vi "stepper controller -- IMS -- V3.vi"(7 "stepper driver action":T3, 8 "internal stepper driver state IMS":T1={"VISA address"="GPIB0::25::INSTR", "stepper motor state"=enum."stopped", "Motor Address"=0, "speed"=0, "target position"=0.0, "current position"=0.0}, 11 "number":dbl format="%#_13g") -> (0 "internal stepper driver state IMS -- OUT":T1={"VISA address"="GPIB0::25::INSTR", "stepper motor state"=enum."stopped", "Motor Address"=0, "speed"=0, "target position"=0.0, "current position"=0.0}, 1 "stepper motor state OUT":T2, 3 "current position":dbl)   [LabVIEW 2018]
uses:
  stepper motor action.ctl
  stepper motor state.ctl
  internal stepper driver state -- IMS.ctl
  Q - not nan -- integer.vi
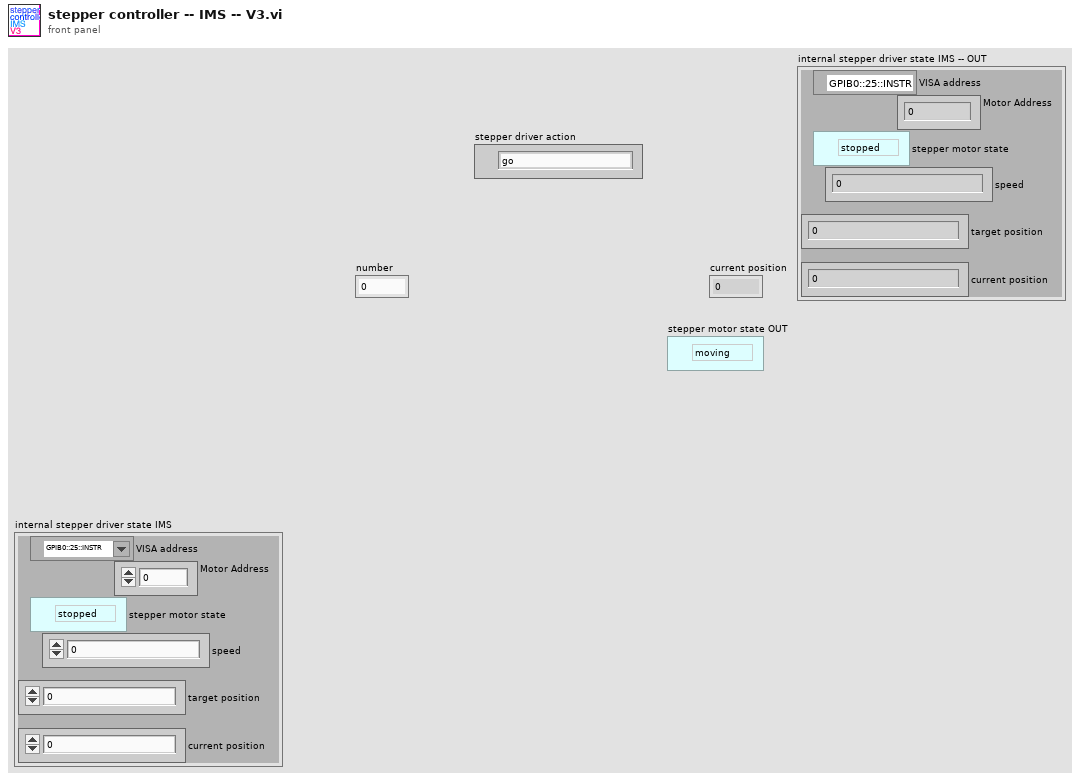
[diagram p1: front panel]
types:
  T1 = typedef "internal stepper driver state -- IMS.ctl" = cluster{"VISA address":refnum<visa-resource-name>, "stepper motor state":T2, "Motor Address":u32, "speed":i32, "target position":dbl, "current position":dbl}
  T2 = typedef "stepper motor state.ctl" = enum16{"moving", "stopped"}
  T3 = typedef "stepper motor action.ctl" = enum16{"go", "void", "stop", "check", "init", "sync", "set", "set speed", "--check status", "--check value"}
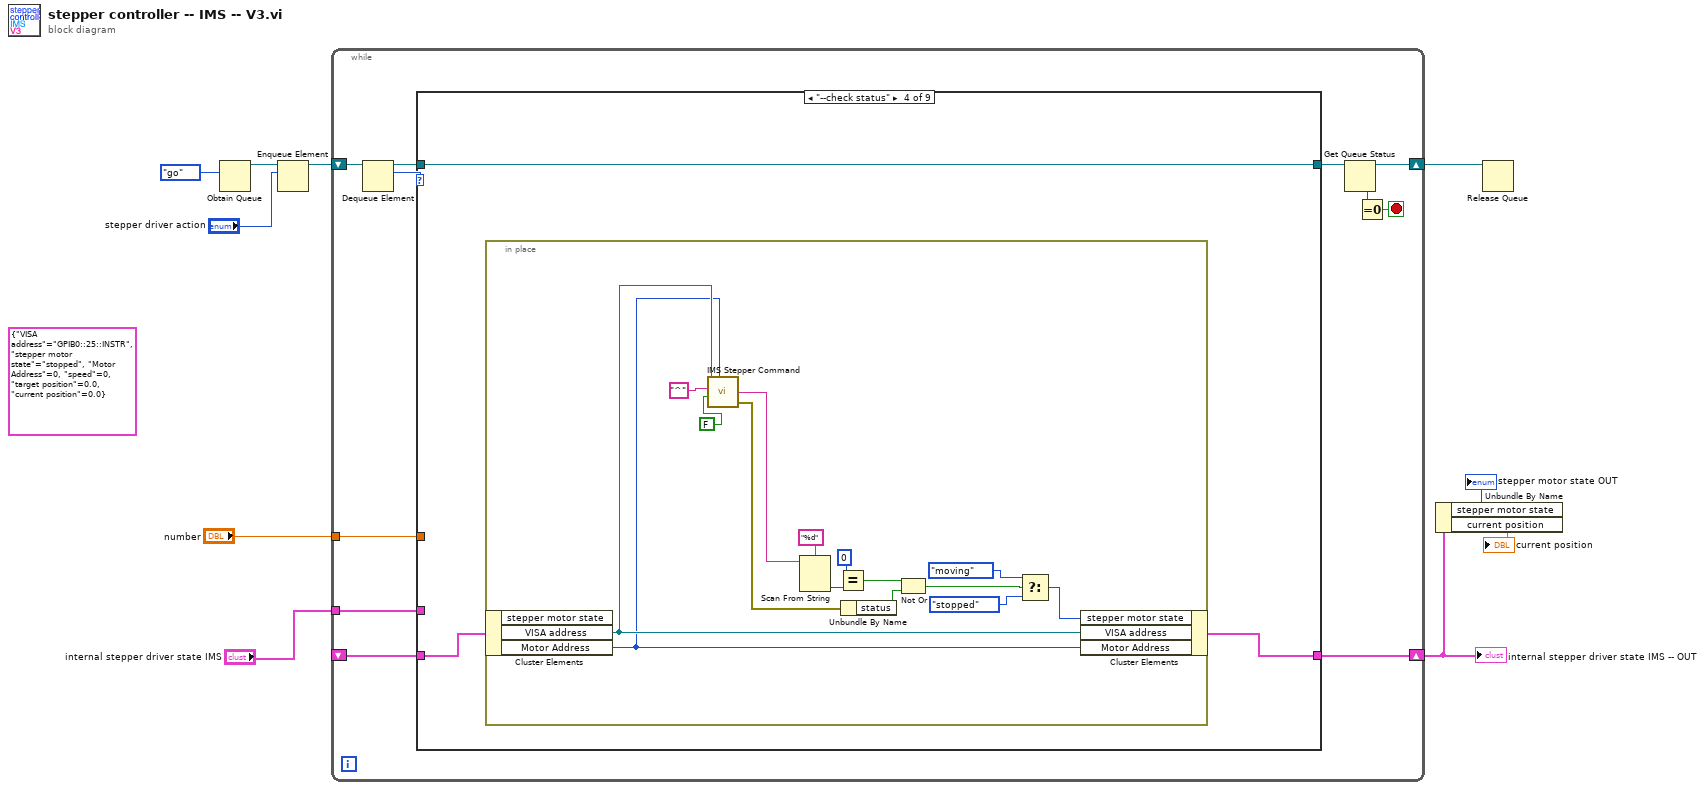
[diagram p0: block diagram]
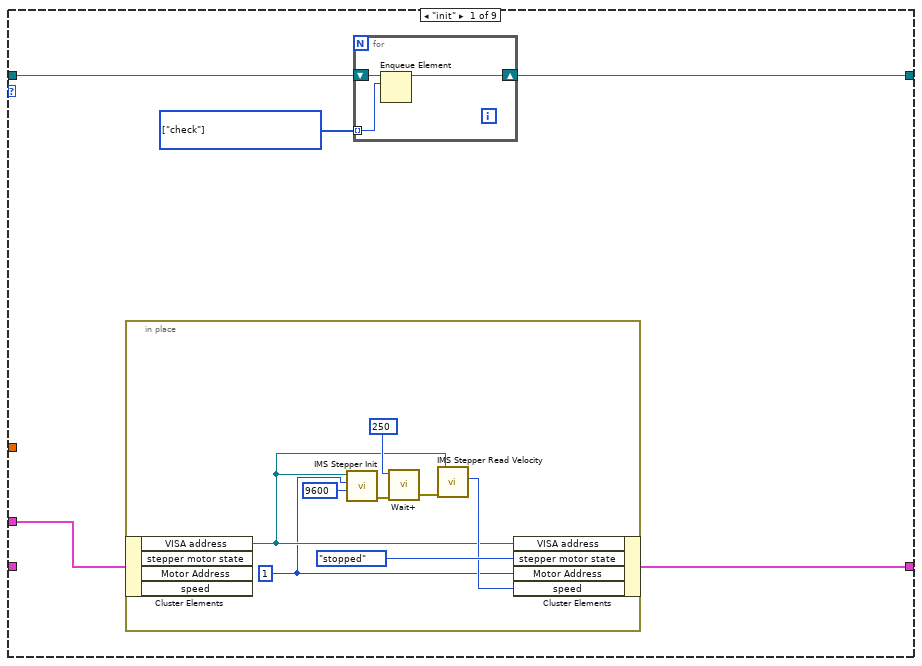
[diagram p2: hidden frame]
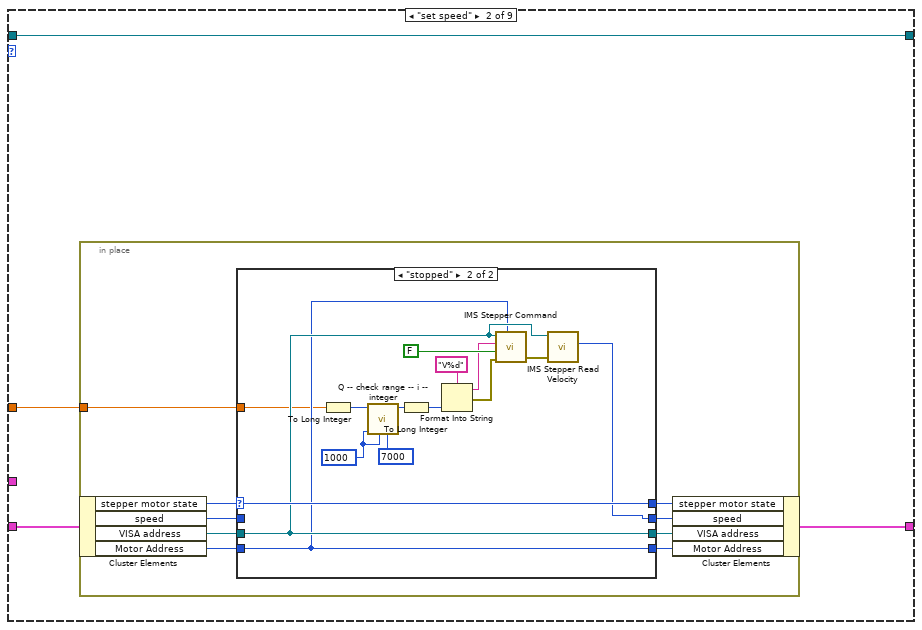
[diagram p3: hidden frame]
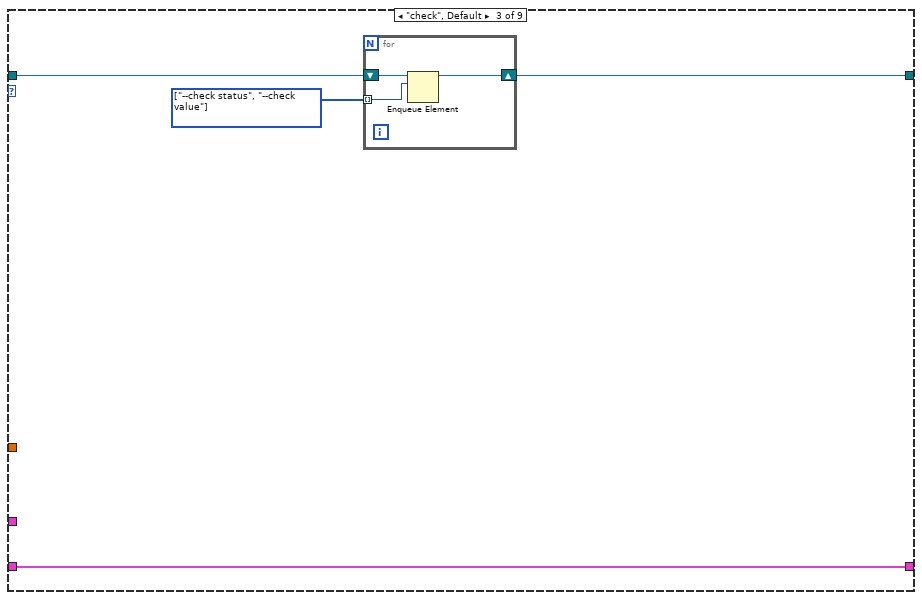
[diagram p5: hidden frame]
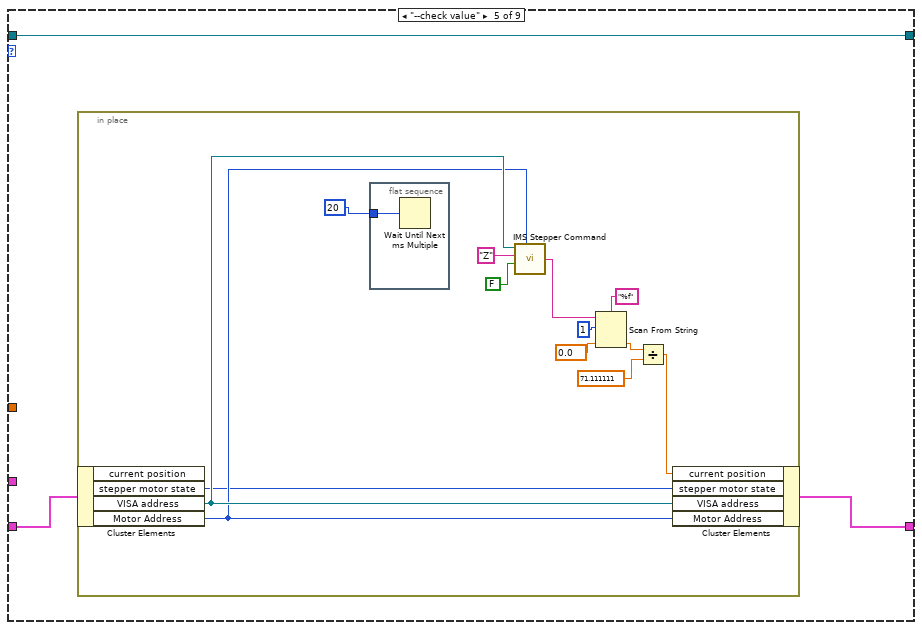
[diagram p6: hidden frame]
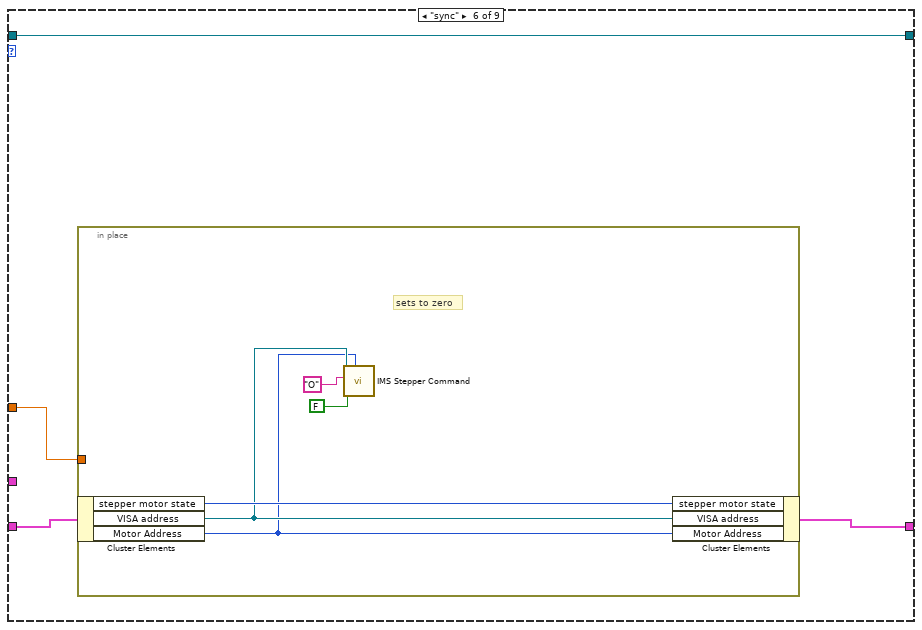
[diagram p7: hidden frame]
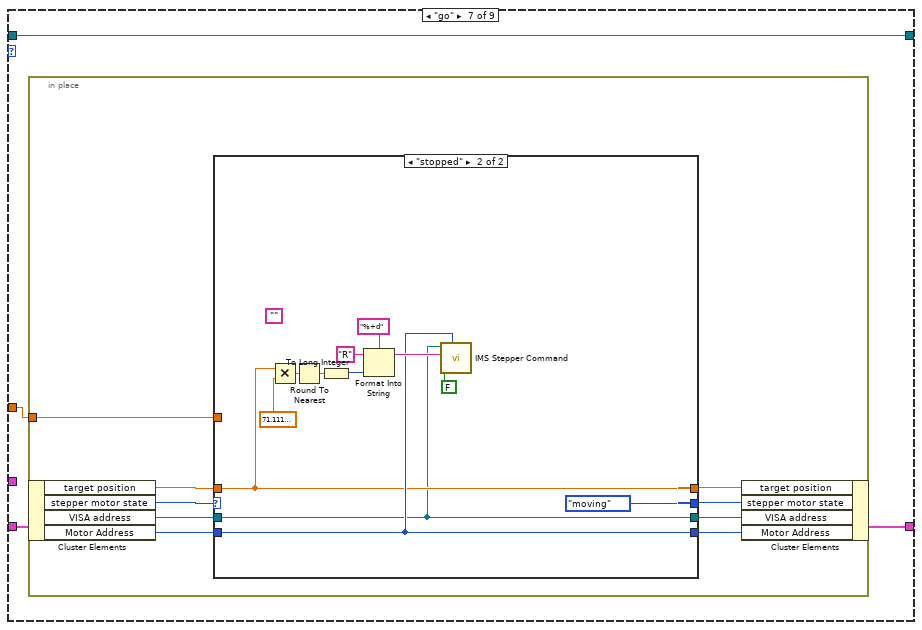
[diagram p8: hidden frame]
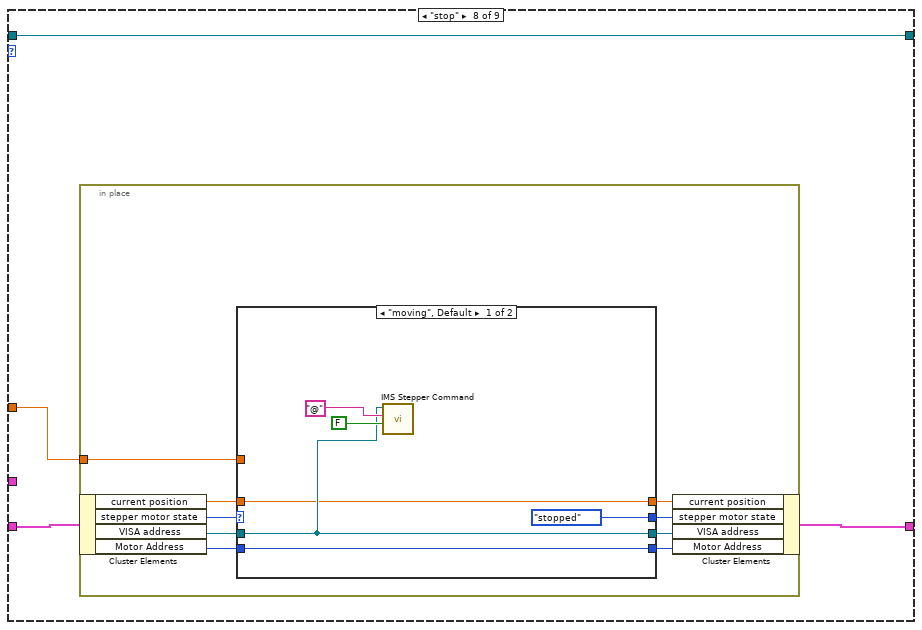
[diagram p10: hidden frame]
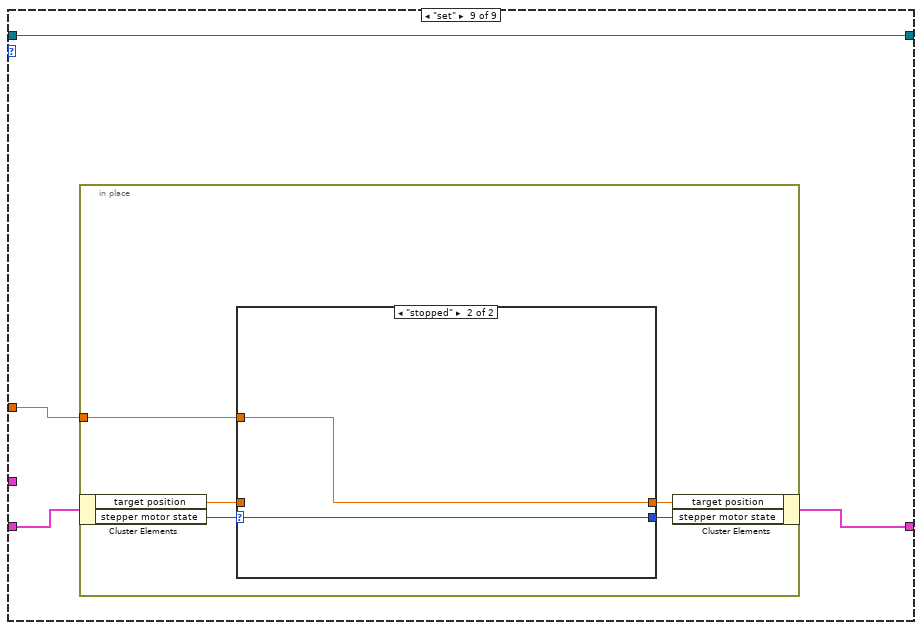
[diagram p12: hidden frame]
diagram:
  (unwired) T1 {"VISA address"="GPIB0::25::INSTR", "stepper motor state"=enum."stopped", "Motor Address"=0, "speed"=0, "target position"=0.0, "current position"=0.0} ("internal stepper driver state IMS")
  n1 = Obtain Queue(element data type=stepper_motor_action."go" ("stepper driver action")) -> (queue out=w4:refnum<queue>)  [unwired: 4 in, 2 out]
  n2 = Enqueue Element(queue=w4, element="stepper driver action") -> (queue out=w3:refnum<queue>)  [unwired: 2 in, 2 out]
  n3 = while {
    shift-right: [w21] -> w6
    shift-left: _ -> [w20]
    shift-right: [w13] -> w1
    shift-left: w3 -> [w17]
    tunnel: "internal stepper driver state IMS" -> [w19]
    tunnel: "number" -> [w18]
    stop <- w11 stop-if-true
    n4 = Dequeue Element(queue=w17) -> (queue out=w16:refnum<queue>, element=w15:T3)  [unwired: 2 in, 2 out]
    n5 = case shown="\"--check status\"" w15 {
      tunnel: [w25 w39 w73 w78 w96 w113 w122 w151 w174] -> w21
      tunnel: w20 -> [_ w40 w73 w79 w97 w114 w123 w152 w175]
      tunnel: [w23 w41 w71 w77 w95 w115 w124 w153 w176] -> w14
      tunnel: w16 -> [w24 w41 w72 w77 w95 w115 w124 w153 w176]
      tunnel: w19 -> [w26 _ _ _ _ _ _ _ _]
      tunnel: w18 -> [_ w38 _ _ _ w112 w121 w150 w173]
      frame "init" {
        w22 = T3[] [enum."check"] items=["go", "void", "stop", "check", "init", "sync", "set", "set speed", "--check status", "--check value"] ("action list IN")
        n6 = in-place {
          w30 = u32 1 ("Motor Address")
          n7 = in-place-cluster #1(w26) -> ("VISA address"=w31:refnum<visa-resource-name>)  [unwired: 3 out]
          n8 = call "IMS Stepper Init.vi"("Baud Rate"=u32 9600, "Motor Number"=w30, "Instrument Address"=w31) -> ("error out"=w36:errorcluster)  [unwired: 1 in, 1 out]
          n9 = call "Wait+.vi"("Error In"=w36, "milliseconds to wait"=u32 250) -> ("Error Out"=w35:errorcluster)  [unwired: 4 in, 1 out]
          n10 = call "IMS Stepper Read Velocity.vi"("error in (no error)"=w35, "Instrument Address"=w31) -> ("Velocity"=w32:i32)  [unwired: 3 in, 2 out]
          n11 = in-place-cluster #1("VISA address"=w31, "stepper motor state"=stepper_motor_state."stopped", "Motor Address"=w30, "speed"=w32) -> (w25:T1)
        }
        n12 = for {
          shift-right: [w28] -> w23
          shift-left: w24 -> [w29]
          tunnel: w22 -> [w27] mode=indexing
          n13 = Enqueue Element(queue=w29, element=w27) -> (queue out=w28:refnum<queue>)  [unwired: 2 in, 2 out]
        }
      }
      frame "set speed" {
        n14 = in-place {
          in-place-border: w38 -> [w50]
          n15 = in-place-cluster #2(w40) -> ("stepper motor state"=w46:T2, "speed"=w45:i32, "VISA address"=w48:refnum<visa-resource-name>, "Motor Address"=w47:u32)
          n16 = case shown="\"stopped\"" w46 {
            selector: w46 -> [w51 w67]
            tunnel: w50 -> [_ w56]
            tunnel: [w54 w58] -> w49
            tunnel: w48 -> [w53 w59]
            tunnel: w47 -> [w52 w57]
            tunnel: w45 -> [w54 _]
            tunnel: [w53 w59] -> w44
            tunnel: [w52 w57] -> w43
            tunnel: [w51 w67] -> w42
            frame "moving", Default {
            }
            frame "stopped" {
              w69 = 1000 ("lower limit")
              n17 = To Long Integer(number=w56) -> (32bit integer=w55:i32)
              n18 = call "Q -- check range -- i -- integer.vi"("upper"=7000 ("x"), "lower"=w69, "default"=w69, "number"=w55) -> ("number in range"=w61:i32)  [unwired: 5 in, 2 out]
              n19 = To Long Integer(number=w61) -> (32bit integer=w60:i32)
              n20 = Format Into String(format string="V%d", w60) -> (resulting string=w64:string, error out=w63:errorcluster)  [unwired: 2 in]
              n21 = call "IMS Stepper Command.vi"("Instrument Address"=w59, "Motor Number"=w57, "Command"=w64, "Mode"=FALSE, "error in (no error)"=w63) -> ("error out"=w62:errorcluster)  [unwired: 1 in, 2 out]
              n22 = call "IMS Stepper Read Velocity.vi"("error in (no error)"=w62, "Instrument Address"=w59) -> ("Velocity"=w58:i32)  [unwired: 3 in, 2 out]
            }
          }
          n23 = in-place-cluster #2("stepper motor state"=w42, "speed"=w49, "VISA address"=w44, "Motor Address"=w43) -> (w39:T1)
        }
      }
      frame "check", Default {
        w70 = T3[] [enum."--check status", enum."--check value"] items=["go", "void", "stop", "check", "init", "sync", "set", "set speed", "--check status", "--check value"] ("action list IN")
        n24 = for {
          shift-right: [w75] -> w71
          shift-left: w72 -> [w76]
          tunnel: w70 -> [w74] mode=indexing
          n25 = Enqueue Element(queue=w76, element=w74) -> (queue out=w75:refnum<queue>)  [unwired: 2 in, 2 out]
        }
      }
      frame "--check status" {
        n26 = in-place {
          n27 = in-place-cluster #3(w79) -> ("VISA address"=w82:refnum<visa-resource-name>, "Motor Address"=w81:u32)  [unwired: 1 out]
          n28 = call "IMS Stepper Command.vi"("Instrument Address"=w82, "Motor Number"=w81, "Command"="^", "Mode"=FALSE) -> ("Response"=w89:string, "error out"=w80:errorcluster)  [unwired: 2 in, 1 out]
          n29 = Scan From String(format string="%d", input string=w89) -> (output 1=w90:i32)  [unwired: 3 in, 3 out]
          n30 = Equal?(x=0, y=w90) -> (x = y?=w91:bool)
          n31 = Unbundle By Name(w80) -> ("status"=w92:bool)
          n32 = Not Or(1:w92, 2:w91) -> (0:w84:bool)
          n33 = Select(t=stepper_motor_state."moving" ("stepper motor state"), s=w84, f=stepper_motor_state."stopped" ("stepper motor state")) -> (s? t:f=w83:T2)
          n34 = in-place-cluster #3("stepper motor state"=w83, "VISA address"=w82, "Motor Address"=w81) -> (w78:T1)
        }
      }
      frame "--check value" {
        n35 = in-place {
          n36 = in-place-cluster #4(w97) -> ("stepper motor state"=w98:T2, "VISA address"=w102:refnum<visa-resource-name>, "Motor Address"=w101:u32)  [unwired: 1 out]
          n37 = flat-sequence {
            tunnel: u32 20 ("millisecond multiple") -> [w111]
            frame #0 {
              n38 = Wait Until Next ms Multiple(millisecond multiple=w111) -> ()  [unwired: 1 out]
            }
          }
          n39 = call "IMS Stepper Command.vi"("Instrument Address"=w102, "Motor Number"=w101, "Command"="Z", "Mode"=FALSE) -> ("Response"=w107:string)  [unwired: 2 in, 2 out]
          n40 = Scan From String(format string="%f", input string=w107, initial scan location=u32 1, default 1=0.0 ("default value 1")) -> (output 1=w109:dbl)  [unwired: 1 in, 3 out]
          n41 = Divide(x=w109, y=71.111111) -> (x/y=w100:dbl)
          n42 = in-place-cluster #4("current position"=w100, "stepper motor state"=w98, "VISA address"=w102, "Motor Address"=w101) -> (w96:T1)
        }
      }
      frame "sync" {
        n43 = in-place {
          in-place-border: w112 -> [_]
          # "sets to zero"
          n44 = in-place-cluster #5(w114) -> ("stepper motor state"=w120:T2, "VISA address"=w117:refnum<visa-resource-name>, "Motor Address"=w116:u32)
          n45 = call "IMS Stepper Command.vi"("Instrument Address"=w117, "Motor Number"=w116, "Command"="O", "Mode"=FALSE) -> ()  [unwired: 2 in, 3 out]
          n46 = in-place-cluster #5("stepper motor state"=w120, "VISA address"=w117, "Motor Address"=w116) -> (w113:T1)
        }
      }
      frame "go" {
        n47 = in-place {
          in-place-border: w121 -> [w133]
          n48 = in-place-cluster #6(w123) -> ("target position"=w127:dbl, "stepper motor state"=w130:T2, "VISA address"=w132:refnum<visa-resource-name>, "Motor Address"=w131:u32)
          n49 = case shown="\"stopped\"" w130 {
            selector: w130 -> [w134 _]
            tunnel: w133 -> [_ _]
            tunnel: w132 -> [w137 w139]
            tunnel: w131 -> [w136 w141]
            tunnel: [w137 w139] -> w129
            tunnel: [w136 w141] -> w128
            tunnel: w127 -> [w135 w140]
            tunnel: [w134 stepper_motor_state."moving" ("stepper motor state")] -> w126
            tunnel: [w135 w140] -> w125
            frame "moving", Default {
            }
            frame "stopped" {
              (unwired) ""
              n50 = Multiply(x=w140, y=71.11111111) -> (x*y=w147:dbl)
              n51 = Round To Nearest(number=w147) -> (nearest integer value=w145:dbl)
              n52 = To Long Integer(number=w145) -> (32bit integer=w146:i32)
              n53 = Format Into String(format string="%+d", initial string="R", w146) -> (resulting string=w142:string)  [unwired: 1 in, 1 out]
              n54 = call "IMS Stepper Command.vi"("Instrument Address"=w139, "Motor Number"=w141, "Command"=w142, "Mode"=FALSE) -> ()  [unwired: 2 in, 3 out]
            }
          }
          n55 = in-place-cluster #6("target position"=w125, "stepper motor state"=w126, "VISA address"=w129, "Motor Address"=w128) -> (w122:T1)
        }
      }
      frame "stop" {
        n56 = in-place {
          in-place-border: w150 -> [w162]
          n57 = in-place-cluster #7(w152) -> ("current position"=w154:dbl, "stepper motor state"=w159:T2, "VISA address"=w161:refnum<visa-resource-name>, "Motor Address"=w160:u32)
          n58 = case shown="\"moving\", Default" w159 {
            selector: w159 -> [_ w170]
            tunnel: w162 -> [_ _]
            tunnel: w161 -> [w164 w172]
            tunnel: w160 -> [w168 w171]
            tunnel: [w164 w172] -> w158
            tunnel: [w168 w171] -> w157
            tunnel: [stepper_motor_state."stopped" ("stepper motor state") w170] -> w156
            tunnel: [w163 w169] -> w155
            tunnel: w154 -> [w163 w169]
            frame "moving", Default {
              n59 = call "IMS Stepper Command.vi"("Instrument Address"=w164, "Command"="@", "Mode"=FALSE) -> ()  [unwired: 3 in, 3 out]
            }
            frame "stopped" {
            }
          }
          n60 = in-place-cluster #7("current position"=w155, "stepper motor state"=w156, "VISA address"=w158, "Motor Address"=w157) -> (w151:T1)
        }
      }
      frame "set" {
        n61 = in-place {
          in-place-border: w173 -> [w181]
          n62 = in-place-cluster #8(w175) -> ("target position"=w177:dbl, "stepper motor state"=w180:T2)
          n63 = case shown="\"stopped\"" w180 {
            selector: w180 -> [w183 w185]
            tunnel: w181 -> [_ w184]
            tunnel: [w183 w185] -> w179
            tunnel: [w182 w184] -> w178
            tunnel: w177 -> [w182 _]
            frame "moving", Default {
            }
            frame "stopped" {
            }
          }
          n64 = in-place-cluster #8("target position"=w178, "stepper motor state"=w179) -> (w174:T1)
        }
      }
    }
    n65 = Get Queue Status(queue=w14) -> (queue out=w13:refnum<queue>, # elements in queue=w12:i32)  [unwired: 2 in, 6 out]
    n66 = Equal To 0?(x=w12) -> (x = 0?=w11:bool)
  }
  "internal stepper driver state IMS -- OUT" <- w6
  n67 = Unbundle By Name(w6) -> ("stepper motor state"=→"stepper motor state OUT":T2, "current position"=→"current position":dbl)
  n68 = Release Queue(queue=w1) -> ()  [unwired: 2 in, 3 out]
